vi "Clear Chart.vi"(8 "error in":errorcluster) -> (0 "error out":errorcluster)   [LabVIEW 2014, in "Chart Module.lvlib"]
uses:
  Chart Module.lvlib
  Clear Chart--arguments.ctl
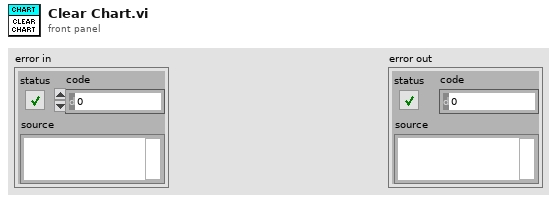
[diagram p1: front panel]
types:
  T1 = typedef "Chart Module.lvlib/Clear Chart--arguments.ctl" = cluster{"Clear Chart?":bool}
  T2 = typedef "Chart Module.lvlib/Request Events--cluster.ctl" = cluster{"Stop Module":refnum<user-event>, "Show Panel":refnum<user-event>, "Hide Panel":refnum<user-event>, "Update Limits":refnum<user-event>, "Send Value":refnum<user-event>, "Clear Chart":refnum<user-event>}
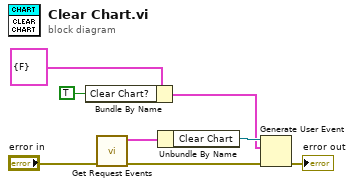
[diagram p0: block diagram]
diagram:
  n1 = Bundle By Name(cluster=T1 {"Clear Chart?"=FALSE} ("Clear Chart Arguments"), "Clear Chart?"=TRUE) -> (w2:T1)
  n2 = call "Get Request Events.vi"("error in"="error in") -> ("error out"=w6:errorcluster, "Request Events"=w8:T2)  [unwired: 9 in]
  n3 = Unbundle By Name(w8) -> ("Clear Chart"=w7:refnum<user-event>)
  n4 = Generate User Event(user event=w7, event data cluster=w2, error in=w6) -> (error out=→"error out":errorcluster)  [unwired: 1 in, 1 out]
